vi "Wheel of Doom Angle to Slot Number.vi"(11 "Sensor Position":dbl) -> (2 "Slot Number":u32, 3 "Normalized Sensor Positon":dbl)   [LabVIEW 2019]
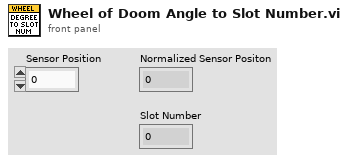
[diagram p1: front panel]
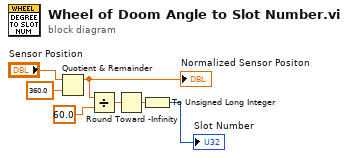
[diagram p0: block diagram]
diagram:
  n1 = Quotient & Remainder(x="Sensor Position", y=360.0) -> (x-y*floor(x/y)=w7:dbl)  [unwired: 1 out]
  "Normalized Sensor Positon" <- w7
  n2 = Divide(x=w7, y=60.0) -> (x/y=w4:dbl)
  n3 = Round Toward -Infinity(1:w4) -> (0:w5:dbl)
  n4 = To Unsigned Long Integer(number=w5) -> (unsigned 32bit integer=→"Slot Number":u32)
